vi "MFLI--init.vi"() -> ()   [LabVIEW 2019]
uses:
  publisher action.ctl
  MFLI frontend action.ctl
panel:
  in  "MFLI Address":string="dev3523"
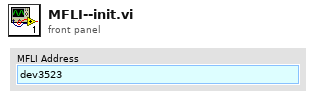
[diagram p1: front panel]
types:
  T1 = typedef "MFLI frontend action.ctl" = enum16{"read", "writeread", "open", "close", "write"}
  T2 = typedef "publisher action.ctl" = enum16{"set", "get", "init", "check"}
  T3 = typedef "Zurich Instruments LabOne.lvlib/ziTypeHandle.ctl" = cluster{"handleValid":bool, "Conn":u64, "Path Prefix":string, "Handle":u64, "Connected":bool, "Clockbase(s)":dbl}
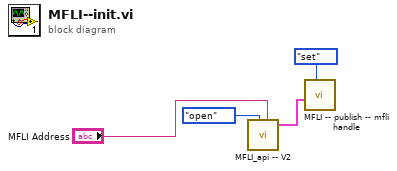
[diagram p0: block diagram]
diagram:
  n1 = call "MFLI_api -- V2.vi"("MFLI Address"="MFLI Address", "MFLI frontend action"=MFLI_frontend_action."open") -> ("Handle Out"=w2:T3)  [unwired: 6 in, 3 out]
  n2 = call "MFLI -- publish -- mfli handle.vi"("publisher action"=publisher_action."set", "Handle IN"=w2) -> ()  [unwired: 9 in, 1 out]
